vi "Read Minimum dt.vi"(11 "error in (no error)":errorcluster) -> (4 "refnum":T1, 6 "File Exist?":bool, 15 "error out":errorcluster)   [LabVIEW 2024, in "devicePowerSequencerCoreLogic.lvlib"]
uses:
  devicePowerSequencerCoreLogic.lvlib
  <vilib>/Utility/config.llb/Config Data RefNum.ctl
  <vilib>/Utility/config.llb/NI_LVConfig.lvlib
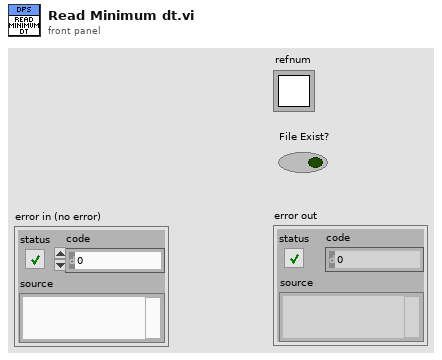
[diagram p1: front panel]
types:
  T1 = typedef "NI_LVConfig.lvlib/Config Data RefNum.ctl" = refnum<k1>
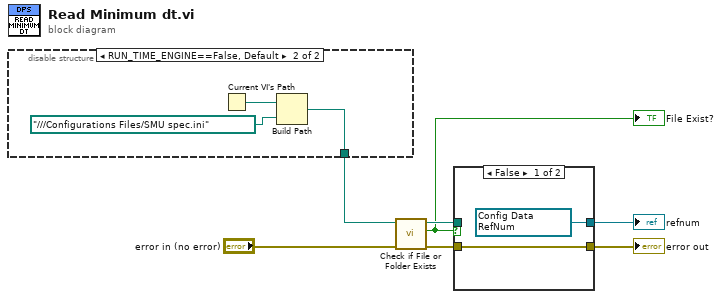
[diagram p0: block diagram]
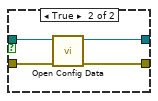
[diagram p2: hidden frame]
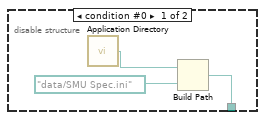
[diagram p3: hidden frame]
diagram:
  n1 = disable-structure shown="RUN_TIME_ENGINE==False, Default" {
    disable-tunnel: [w8 w11] -> w5
    frame condition #0 {
      n2 = call <vilib>:"Application Directory.vi"() -> ("Application Directory"=w10:path)
      n3 = Build Path(base path=w10, name or relative path=path "data/SMU Spec.ini") -> (appended path=w8:path)
    }
    frame condition #1 (active) {
      n4 = Current VI's Path() -> (path=w13:path)
      n5 = Build Path(base path=w13, name or relative path=path "../../../Configurations Files/SMU spec.ini") -> (appended path=w11:path)
    }
  }
  n6 = call <vilib>:"Check if File or Folder Exists.vi"("error in (no error)"="error in (no error)", "path"=w5) -> ("error out"=w4:errorcluster, "file or folder exists?"=w1:bool, "dup path"=w2:path)  [unwired: 7 in]
  "File Exist?" <- w1
  n7 = case shown="False" w1 {
    tunnel: [w14 w19] -> w7
    tunnel: [w15 w18] -> w6
    tunnel: w4 -> [w14 w17]
    tunnel: w2 -> [_ w16]
    frame False {
      w15 = T1 refnum items=["config data"] ("refnum")
    }
    frame True {
      n8 = call <vilib>:"Open Config Data.vi"("error in (no error)"=w17, "configuration file path"=w16) -> ("error out"=w19:errorcluster, "refnum"=w18:T1)  [unwired: 7 in, 1 out]
    }
  }
  "error out" <- w7
  "refnum" <- w6
